vi "Analysis.LevelTransition.ODH.vi"(9 "Numeric":dbl, 10 "LVTransitionParameters":T1, 11 "Array in":dbl[][](array[numeric])) -> (2 "Results":dbl[](array[numeric]), 3 "Array out":bool[](array[boolean]))   [LabVIEW 2015, in "TestStand Analysis Steps.lvlib"]
uses:
  TestStand Analysis Steps.lvlib
  Shared/Public.LVAnalysis.ctl
  Shared/Public.ChLVAnalysis.ctl
  Shared/Shared.lvlib
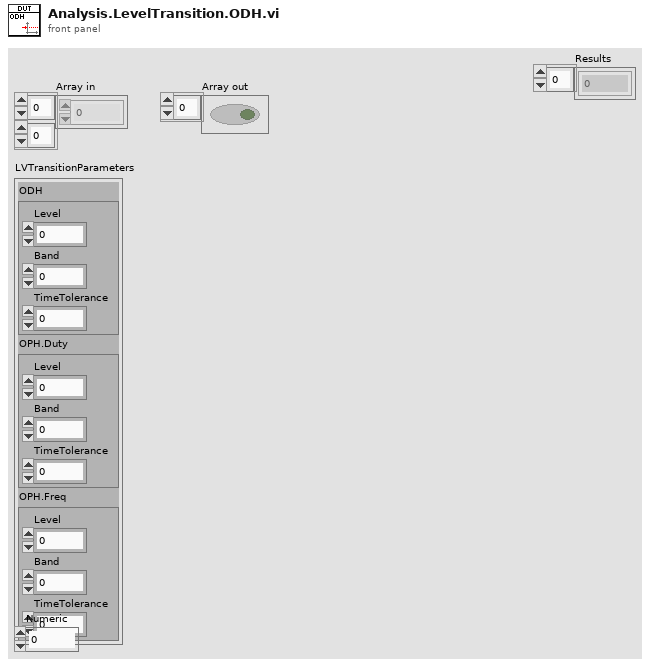
[diagram p1: front panel]
types:
  T1 = typedef "Shared.lvlib/Public.LVAnalysis.ctl" = cluster{"ODH":T2, "OPH.Duty":T2, "OPH.Freq":T2}
  T2 = typedef "Shared.lvlib/Public.ChLVAnalysis.ctl" = cluster{"Level":dbl, "Band":dbl, "TimeTolerance":dbl}
  T3 = cluster{"Scale":dbl, "Hi":dbl, "Lo":dbl, "dt":dbl, "Timeout":dbl}
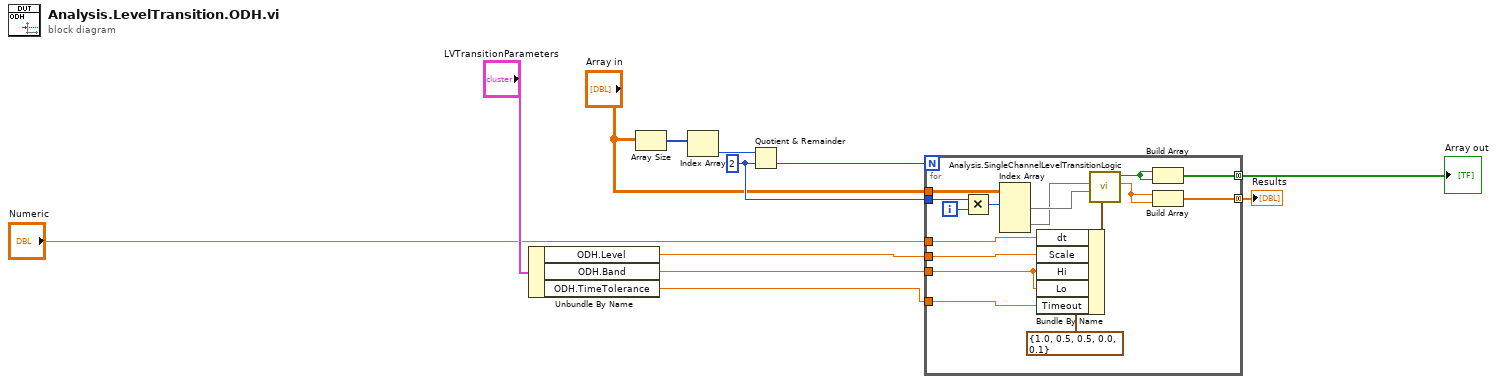
[diagram p0: block diagram]
diagram:
  w6 = 2 ("y")
  n1 = Unbundle By Name("LVTransitionParameters") -> ("ODH.Level"=w9:dbl, "ODH.Band"=w10:dbl, "ODH.TimeTolerance"=w11:dbl)
  n2 = Array Size(array="Array in") -> (size(s)=w3:i32[])
  n3 = Index Array(array=w3) -> (element=w4:i32)  [unwired: 1 in]
  n4 = Quotient & Remainder(x=w4, y=w6) -> (floor(x/y)=w5:i32)  [unwired: 1 out]
  n5 = for {
    N: w5 -> [_]
    tunnel: "Array in" -> [w28]
    tunnel: w6 -> [w21]
    tunnel: [w19] -> w7 mode=concatenating
    tunnel: "Numeric" -> [w18]
    tunnel: w9 -> [w17]
    tunnel: w10 -> [w16]
    tunnel: w11 -> [w15]
    tunnel: [w13] -> w1 mode=concatenating
    i -> [w23]
    n6 = Multiply(x=w21, y=w23) -> (x*y=w22:i32)
    n7 = Index Array(array=w28, index (row) #1=w22) -> (element #1=w25:dbl[], element #2=w24:dbl[])  [unwired: 3 in]
    n8 = Bundle By Name(cluster=T3 {"Scale"=1.0, "Hi"=0.5, "Lo"=0.5, "dt"=0.0, "Timeout"=0.1} ("Parameters"), "dt"=w18, "Scale"=w17, "Hi"=w16, "Lo"=w16, "Timeout"=w15) -> (w26:T3)
    n9 = call "Analysis.SingleChannelLevelTransitionLogic.vi"("Stimulus"=w25, "Response"=w24, "Parameters"=w26) -> ("Result"=w14:dbl, "Fail"=w20:bool)  [unwired: 7 in]
    n10 = Build Array(w20, w20) -> (w19:bool[])
    n11 = Build Array(w14, w14) -> (w13:dbl[])
  }
  "Array out" <- w7
  "Results" <- w1
